vi "p1.vi"() -> ()   [LabVIEW 2021, in "d1.lvlib"]
uses:
  d1.lvlib
  AOC/AOC.lvlib
panel:
  in  "Example":string="1000\n2000\n3000\n\n4000\n\n5000\n6000\n\n7000\n8000\n9000\n\n10000\n"
  in  "Example?":bool
  out "Answer":i32=71934
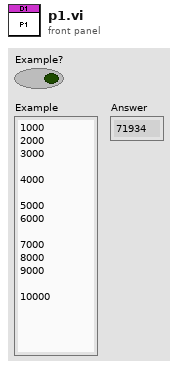
[diagram p1: front panel]
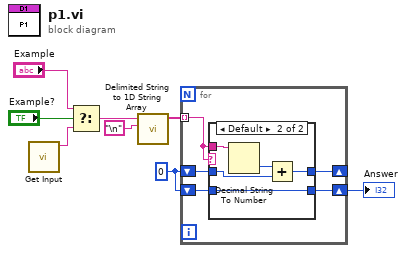
[diagram p0: block diagram]
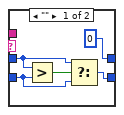
[diagram p2: hidden frame]
diagram:
  w1 = 0
  n1 = call "Get Input.vi"() -> ("Input"=w6:string)  [unwired: 11 in]
  n2 = Select(t="Example", s="Example?", f=w6) -> (s? t:f=w4:string)
  n3 = call <vilib>:"Delimited String to 1D String Array.vi"("delimiter"="\n", "delimited string"=w4) -> ("string array"=w3:string[])  [unwired: 9 in]
  n4 = for {
    tunnel: w3 -> [w11] mode=indexing
    shift-right: [w13] -> _
    shift-left: w1 -> [w12]
    shift-right: [w10] -> w8
    shift-left: w1 -> [w9]
    n5 = case shown="Default" w11 {
      tunnel: [0 w23] -> w13
      tunnel: w12 -> [w14 w22]
      tunnel: w11 -> [_ w20]
      tunnel: [w15 w19] -> w10
      tunnel: w9 -> [w16 w19]
      frame "" {
        n6 = Greater?(x=w14, y=w16) -> (0:w17:bool)
        n7 = Select(t=w14, s=w17, f=w16) -> (s? t:f=w15:i32)
      }
      frame Default {
        n8 = Decimal String To Number(string=w20) -> (number=w21:i32)  [unwired: 2 in, 1 out]
        n9 = Add(x=w21, y=w22) -> (x+y=w23:i32)
      }
    }
  }
  "Answer" <- w8
